vi "ziAutoRange.vi"(8 "Error in":errorcluster, 10 "Path":string, 11 "Handle in":T1 {"Handle" format="0x%08x"; "Conn" format="0x%08x"}) -> (0 "Error out":errorcluster, 1 "Success":bool, 3 "Handle out":T1 {"Handle" format="0x%08x"; "Conn" format="0x%08x"})   [LabVIEW 2015, in "Zurich Instruments LabOne.lvlib"]
doc: "Automatically set the input range of signalinputs/{0,1} to half full level.\n<B>Path</B> can either be sigins/0 or sigins/1"
uses:
  Zurich Instruments LabOne.lvlib
  ziTypeHandle.ctl
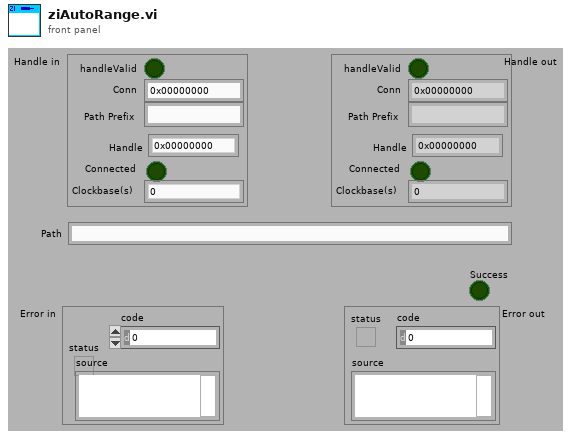
[diagram p1: front panel]
types:
  T1 = typedef "Zurich Instruments LabOne.lvlib/ziTypeHandle.ctl" = cluster{"handleValid":bool, "Conn":u64, "Path Prefix":string, "Handle":u64, "Connected":bool, "Clockbase(s)":dbl}
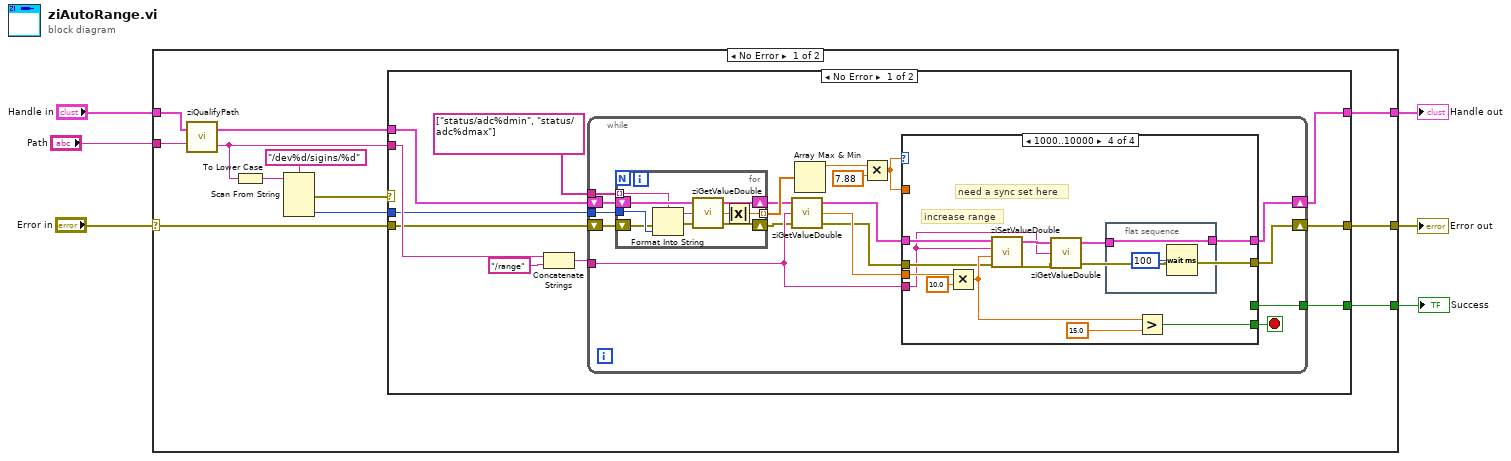
[diagram p0: block diagram]
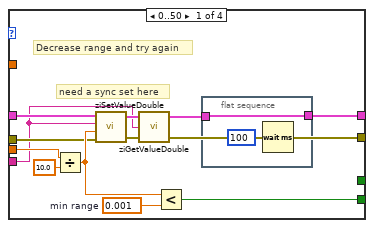
[diagram p2: hidden frame]
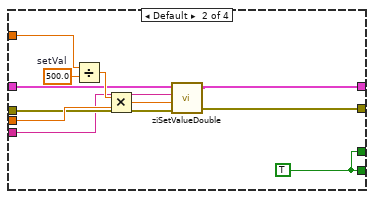
[diagram p3: hidden frame]
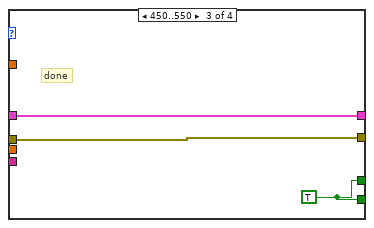
[diagram p4: hidden frame]
diagram:
  n1 = case shown="No Error" "Error in" {
    selector: "Error in" -> [w16 w103]
    tunnel: [w18 w103] -> w6
    tunnel: [w17 w104] -> w5
    tunnel: "Handle in" -> [w14 w104]
    tunnel: "Path" -> [w15 _]
    tunnel: [w10 _] -> w1
    frame No Error {
      n2 = call "ziQualifyPath.vi"("Path In"=w15, "Handle In"=w14) -> ("Path Out"=w9:string, "Handle Out"=w13:T1)
      n3 = To Lower Case(string=w9) -> (all lower case string=w8:string)
      n4 = Scan From String(format string="/dev%d/sigins/%d" ("regular expression"), input string=w8) -> (error out=w12:errorcluster, output 2=w7:i32)  [unwired: 5 in, 2 out]
      n5 = case shown="No Error" w12 {
        tunnel: [w25 w102] -> w18
        tunnel: [w26 w101] -> w17
        tunnel: w13 -> [w27 w101]
        tunnel: w16 -> [w19 w102]
        tunnel: w9 -> [w22 _]
        tunnel: w7 -> [w20 _]
        tunnel: [w21 _] -> w10
        frame No Error {
          n6 = Concatenate Strings(w22, "/range") -> (w24:string)
          n7 = while {
            shift-right: [w43] -> w26
            shift-left: w27 -> [w39]
            shift-right: [w42] -> w25
            shift-left: w19 -> [w31]
            tunnel: w24 -> [w34]
            tunnel: string[] ["status/adc%dmin", "status/adc%dmax"] -> [w38]
            tunnel: w20 -> [w30]
            tunnel: [w29] -> w21
            stop <- w41 stop-if-true
            n8 = for {
              tunnel: w38 -> [w51] mode=indexing
              tunnel: [w56] -> w46 mode=indexing
              shift-right: [w55] -> w37
              shift-left: w39 -> [w54]
              tunnel: w30 -> [w50]
              shift-right: [w52] -> w32
              shift-left: w31 -> [w48]
              n9 = Format Into String(format string=w51, error in=w48, w50) -> (resulting string=w49:string, error out=w47:errorcluster)  [unwired: 1 in]
              n10 = call "ziGetValueDouble.vi"("error in"=w47, "Path"=w49, "Handle in"=w54) -> ("error out"=w52:errorcluster, "Value"=w53:dbl, "Handle out"=w55:T1)
              n11 = Absolute Value(x=w53) -> (abs(x)=w56:dbl)
            }
            n12 = call "ziGetValueDouble.vi"("error in"=w32, "Path"=w34, "Handle in"=w37) -> ("error out"=w33:errorcluster, "Value"=w35:dbl, "Handle out"=w36:T1)
            n13 = Array Max & Min(array=w46) -> (max value=w44:dbl)  [unwired: 3 out]
            n14 = Multiply(x=w44, y=7.88 ("valueD")) -> (x*y=w40:dbl)
            n15 = case shown="1000..10000" w40 {
              tunnel: w36 -> [w66 w76 w84 w94]
              tunnel: w33 -> [w64 w74 w85 w92]
              tunnel: [w59 w78 w84 w88] -> w43
              tunnel: [w58 w77 w85 w87] -> w42
              tunnel: [w57 w72 w83 w95] -> w41
              tunnel: w35 -> [w69 w82 _ w97]
              tunnel: w40 -> [_ w80 _ _]
              tunnel: w34 -> [w62 w73 _ w86]
              tunnel: [_ w72 w83 _] -> w29
              frame 0..50 {
                w67 = 0.001  # min range
                # "need a sync set here"
                # "Decrease range and try again"
                n16 = Divide(x=w69, y=10.0 ("valueD")) -> (x/y=w65:dbl)
                n17 = call "ziSetValueDouble.vi"("Error In"=w64, "Value"=w65, "Path"=w62, "Handle In"=w66) -> ("Error Out"=w61:errorcluster, "Handle Out"=w63:T1)  [unwired: 1 in]
                n18 = call "ziGetValueDouble.vi"("error in"=w61, "Path"=w62, "Handle in"=w63) -> ("error out"=w58:errorcluster, "Handle out"=w60:T1)  [unwired: 1 out]
                n19 = Less?(x=w65, y=w67) -> (x < y?=w57:bool)
                n20 = flat-sequence {
                  tunnel: w60 -> [w70]
                  tunnel: [w70] -> w59
                  frame #0 {
                    n21 = Wait (ms)(milliseconds to wait=u32 100) -> ()  [unwired: 1 out]
                  }
                }
              }
              frame Default {
                w79 = 500.0  # setVal
                w72 = TRUE
                n22 = Divide(x=w80, y=w79) -> (x/y=w81:dbl)
                n23 = Multiply(x=w81, y=w82) -> (x*y=w75:dbl)
                n24 = call "ziSetValueDouble.vi"("Error In"=w74, "Value"=w75, "Path"=w73, "Handle In"=w76) -> ("Error Out"=w77:errorcluster, "Handle Out"=w78:T1)  [unwired: 1 in]
              }
              frame 450..550 {
                w83 = TRUE
                # "done"
              }
              frame 1000..10000 {
                # "need a sync set here"
                # "increase range"
                n25 = Multiply(x=w97, y=10.0 ("valueD")) -> (x*y=w93:dbl)
                n26 = call "ziSetValueDouble.vi"("Error In"=w92, "Value"=w93, "Path"=w86, "Handle In"=w94) -> ("Error Out"=w90:errorcluster, "Handle Out"=w91:T1)  [unwired: 1 in]
                n27 = call "ziGetValueDouble.vi"("error in"=w90, "Path"=w86, "Handle in"=w91) -> ("error out"=w87:errorcluster, "Handle out"=w89:T1)  [unwired: 1 out]
                n28 = flat-sequence {
                  tunnel: w89 -> [w99]
                  tunnel: [w99] -> w88
                  frame #0 {
                    n29 = Wait (ms)(milliseconds to wait=u32 100) -> ()  [unwired: 1 out]
                  }
                }
                n30 = Greater?(x=w93, y=15.0 ("valueD")) -> (0:w95:bool)
              }
            }
          }
        }
        frame Error {
        }
      }
    }
    frame Error {
    }
  }
  "Handle out" <- w5
  "Error out" <- w6
  "Success" <- w1
